vi "get_com_port.vi"(8 "error in (no error)":errorcluster, 11 "StageMH110930Scientifica in":refnum<class "StageMMS2015ASIfromScientifica.lvclass">) -> (0 "error out":errorcluster, 2 "serial port name":refnum<visa-resource-name>, 3 "StageMH110930Scientifica out":refnum<class "StageMMS2015ASIfromScientifica.lvclass">)   [LabVIEW 2010, in "StageMMS2015ASIfromScientifica.lvclass"]
uses:
  StageMMS2015ASIfromScientifica.lvclass
  StageMMS2015ASIfromScientifica.lvclass/StageMMS2015ASIfromScientifica.ctl
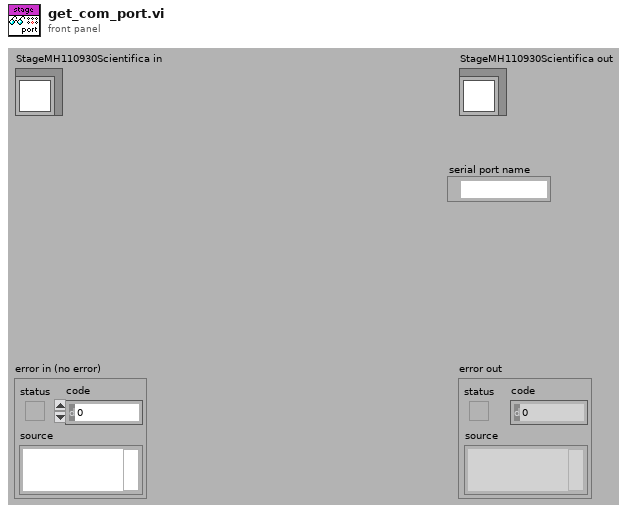
[diagram p1: front panel]
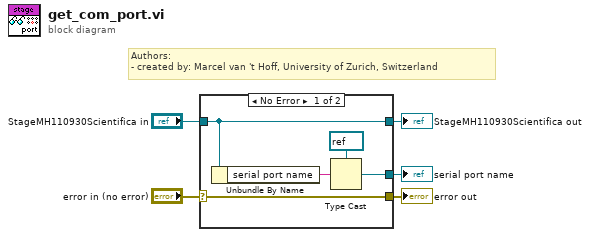
[diagram p0: block diagram]
diagram:
  # "Authors: \n- created by: Marcel van 't Hoff, University of Zurich, Switzerland"
  n1 = case shown="No Error" "error in (no error)" {
    selector: "error in (no error)" -> [w10 w12]
    tunnel: [w10 w12] -> w4
    tunnel: [w9 w11] -> w2
    tunnel: "StageMH110930Scientifica in" -> [w9 w11]
    tunnel: [w7 _] -> w1
    frame No Error {
      n2 = Unbundle By Name(w9) -> ("serial port name"=w8:string)
      n3 = Type Cast(type=refnum<visa-resource-name> refnum ("serial port name"), x=w8) -> (*(type *) &x=w7:refnum<visa-resource-name>)
    }
    frame Error {
    }
  }
  "error out" <- w4
  "StageMH110930Scientifica out" <- w2
  "serial port name" <- w1
